vi "Execute Job (Async).vi"(6 "timeout (500 ms)":i32=500, 8 "error in (no error)":errorcluster, 10 "stdin":string, 11 "Job in":refnum<class "Job.lvclass">) -> (0 "error out":errorcluster, 2 "Job GUID":string, 3 "Job out":refnum<class "Job.lvclass">)   [LabVIEW 2013, in "openCronJob.lvlib" / "Job.lvclass"]
uses:
  Job.lvclass
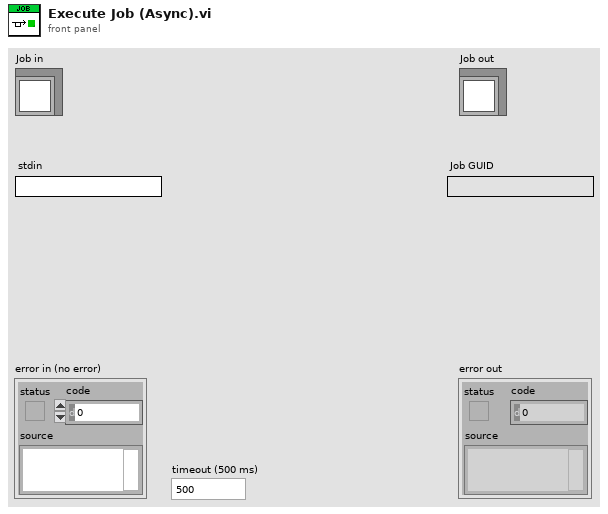
[diagram p1: front panel]
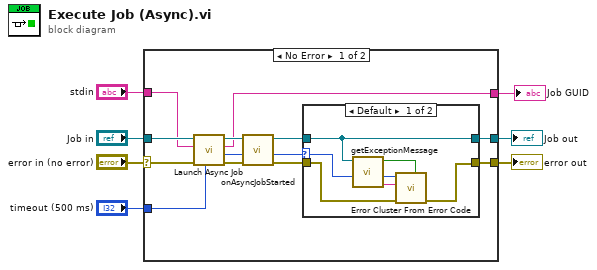
[diagram p0: block diagram]
diagram:
  n1 = case shown="No Error" "error in (no error)" {
    selector: "error in (no error)" -> [w12 w31]
    tunnel: "Job in" -> [w11 w30]
    tunnel: [w14 w30] -> w6
    tunnel: [w13 w31] -> w5
    tunnel: [w10 _] -> w3
    tunnel: "timeout (500 ms)" -> [w9 _]
    tunnel: "stdin" -> [w8 _]
    frame No Error {
      n2 = call "Launch Async Job.vi"("timeout (500 ms)"=w9, "error in (no error)"=w12, "stdin"=w8, "Job in"=w11) -> ("error out"=w18:errorcluster, "exception"=w20:i32, "Job GUID"=w10:string, "Job out"=w19:refnum<class "Job.lvclass">)  [unwired: 4 in]
      n3 = call-dynamic "onAsyncJobStarted.vi"("error in (no error)"=w18, "exception"=w20, "Job in"=w19) -> ("error out"=w16:errorcluster, "unhandled exception"=w17:i32, "Job out"=w15:refnum<class "Job.lvclass">)  [unwired: 6 in]
      n4 = case shown="Default" w17 {
        selector: w17 -> [w25 _]
        tunnel: w16 -> [w27 w28]
        tunnel: w15 -> [w23 w29]
        tunnel: [w23 w29] -> w14
        tunnel: [w26 w28] -> w13
        frame Default {
          n5 = call-dynamic "getExceptionMessage.vi"("exception"=w25, "Job in"=w23) -> ("exception message"=w22:string, "exception dup"=w24:i32, "warning?"=w21:bool)  [unwired: 7 in]
          n6 = call <vilib>:"Error Cluster From Error Code.vi"("is warning? (False)"=w21, "error in (no error)"=w27, "error message (\"\")"=w22, "error code (0)"=w24) -> ("error out"=w26:errorcluster)  [unwired: 5 in]
        }
        frame 0 {
        }
      }
    }
    frame Error {
    }
  }
  "error out" <- w5
  "Job out" <- w6
  "Job GUID" <- w3
